vi "Transform Triangle.vi"(6 "Translation Matrix":sgl[][](array[numeric]), 8 "Rotation Z Matrix":sgl[][](array[numeric]), 9 "Rotation Y Matrix":sgl[][](array[numeric]), 10 "Rotation X Matrix":sgl[][](array[numeric]), 11 "Triangle in":T1={"Vertex 1"={"Position"={"x"=0.0, "y"=0.0, "z"=0.0}, "UV"={"u"=0.0, "v"=0.0}, "Colour"=12517256}, "Vertex 2"={"Position"={"x"=0.0, "y"=0.0, "z"=0.0}, "UV"={"u"=0.0, "v"=0.0}, "Colour"=12517256}, "Vertex 3"={"Position"={"x"=0.0, "y"=0.0, "z"=0.0}, "UV"={"u"=0.0, "v"=0.0}, "Colour"=12517256}, "Alpha"=0.0, "Alpha Blending Enabled"=FALSE} {"Vertex 3"."UV"."v" min=0 max=1 step=0.1; "Vertex 3"."UV"."u" min=0 max=1 step=0.1; "Vertex 2"."UV"."v" min=0 max=1 step=0.1; "Vertex 2"."UV"."u" min=0 max=1 step=0.1; "Vertex 1"."UV"."v" min=0 max=1 step=0.1; "Vertex 1"."UV"."u" min=0 max=1 step=0.1}) -> (3 "Triangle out":T1={"Vertex 1"={"Position"={"x"=0.0, "y"=0.0, "z"=0.0}, "UV"={"u"=0.0, "v"=0.0}, "Colour"=12517256}, "Vertex 2"={"Position"={"x"=0.0, "y"=0.0, "z"=0.0}, "UV"={"u"=0.0, "v"=0.0}, "Colour"=12517256}, "Vertex 3"={"Position"={"x"=0.0, "y"=0.0, "z"=0.0}, "UV"={"u"=0.0, "v"=0.0}, "Colour"=12517256}, "Alpha"=0.0, "Alpha Blending Enabled"=FALSE} {"Vertex 3"."UV"."v" min=0 max=1 step=0.1; "Vertex 3"."UV"."u" min=0 max=1 step=0.1; "Vertex 2"."UV"."v" min=0 max=1 step=0.1; "Vertex 2"."UV"."u" min=0 max=1 step=0.1; "Vertex 1"."UV"."v" min=0 max=1 step=0.1; "Vertex 1"."UV"."u" min=0 max=1 step=0.1})   [LabVIEW 2022 SP3, in "3D.lvlib"]
uses:
  3D.lvlib
  Vector 3D.ctl
  Raster/UV.ctl
  Raster/Raster.lvlib
  Vertex.ctl
  Triangle.ctl
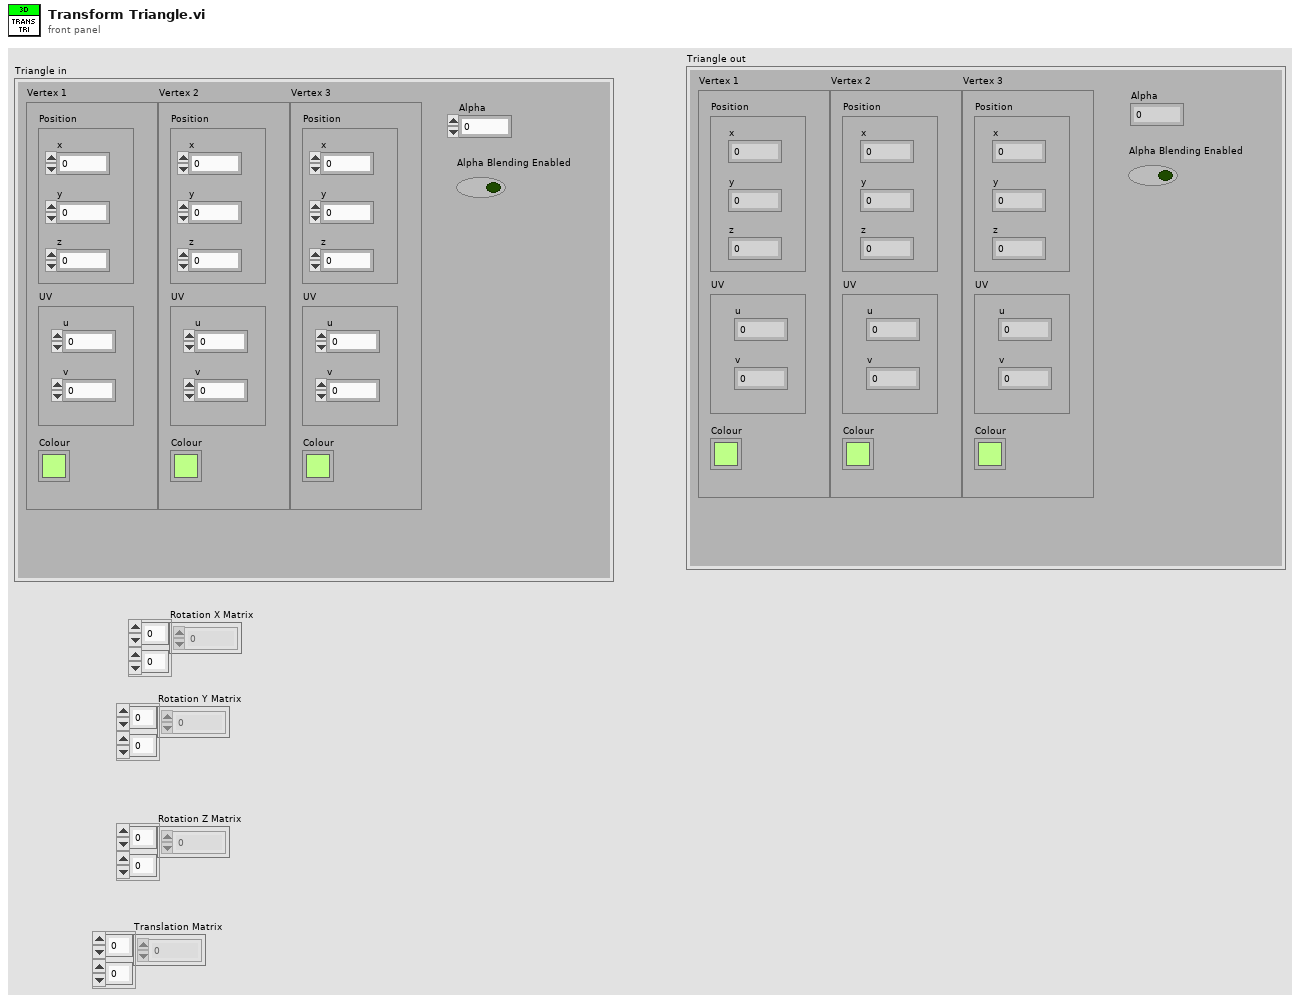
[diagram p1: front panel]
types:
  T1 = typedef "3D.lvlib/Triangle.ctl" = cluster{"Vertex 1":T2, "Vertex 2":T2, "Vertex 3":T2, "Alpha":dbl, "Alpha Blending Enabled":bool}
  T2 = typedef "3D.lvlib/Vertex.ctl" = cluster{"Position":T3, "UV":T4, "Colour":u32}
  T3 = typedef "3D.lvlib/Vector 3D.ctl" = cluster{"x":sgl, "y":sgl, "z":sgl}
  T4 = typedef "Raster.lvlib/UV.ctl" = cluster{"u":sgl, "v":sgl}
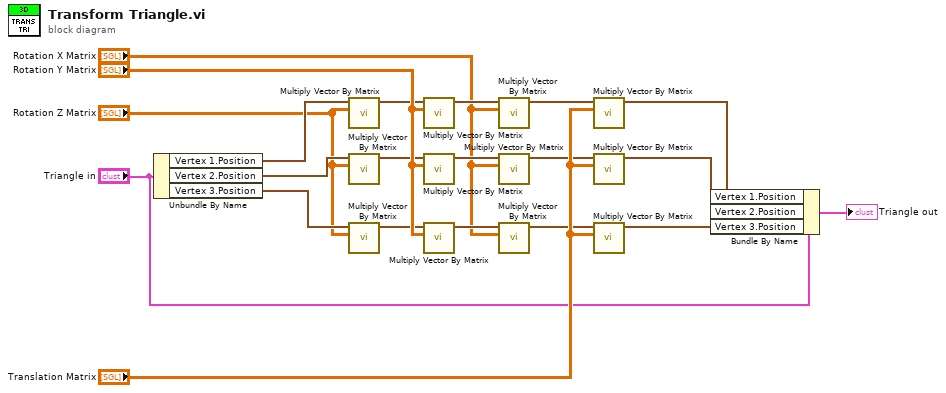
[diagram p0: block diagram]
diagram:
  n1 = Unbundle By Name("Triangle in") -> ("Vertex 1.Position"=w7:T3, "Vertex 2.Position"=w8:T3, "Vertex 3.Position"=w9:T3)
  n2 = call "Multiply Vector By Matrix.vi"("Matrix in"="Rotation Z Matrix", "Vector 3D in"=w7) -> ("Vector 3D out"=w10:T3)  [unwired: 9 in]
  n3 = call "Multiply Vector By Matrix.vi"("Matrix in"="Rotation Z Matrix", "Vector 3D in"=w8) -> ("Vector 3D out"=w12:T3)  [unwired: 9 in]
  n4 = call "Multiply Vector By Matrix.vi"("Matrix in"="Rotation Z Matrix", "Vector 3D in"=w9) -> ("Vector 3D out"=w14:T3)  [unwired: 9 in]
  n5 = call "Multiply Vector By Matrix.vi"("Matrix in"="Rotation Y Matrix", "Vector 3D in"=w10) -> ("Vector 3D out"=w11:T3)  [unwired: 9 in]
  n6 = call "Multiply Vector By Matrix.vi"("Matrix in"="Rotation Y Matrix", "Vector 3D in"=w12) -> ("Vector 3D out"=w13:T3)  [unwired: 9 in]
  n7 = call "Multiply Vector By Matrix.vi"("Matrix in"="Rotation Y Matrix", "Vector 3D in"=w14) -> ("Vector 3D out"=w15:T3)  [unwired: 9 in]
  n8 = call "Multiply Vector By Matrix.vi"("Matrix in"="Rotation X Matrix", "Vector 3D in"=w11) -> ("Vector 3D out"=w4:T3)  [unwired: 9 in]
  n9 = call "Multiply Vector By Matrix.vi"("Matrix in"="Rotation X Matrix", "Vector 3D in"=w13) -> ("Vector 3D out"=w5:T3)  [unwired: 9 in]
  n10 = call "Multiply Vector By Matrix.vi"("Matrix in"="Rotation X Matrix", "Vector 3D in"=w15) -> ("Vector 3D out"=w6:T3)  [unwired: 9 in]
  n11 = call "Multiply Vector By Matrix.vi"("Matrix in"="Translation Matrix", "Vector 3D in"=w4) -> ("Vector 3D out"=w19:T3)  [unwired: 9 in]
  n12 = call "Multiply Vector By Matrix.vi"("Matrix in"="Translation Matrix", "Vector 3D in"=w5) -> ("Vector 3D out"=w20:T3)  [unwired: 9 in]
  n13 = call "Multiply Vector By Matrix.vi"("Matrix in"="Translation Matrix", "Vector 3D in"=w6) -> ("Vector 3D out"=w21:T3)  [unwired: 9 in]
  n14 = Bundle By Name(cluster="Triangle in", "Vertex 1.Position"=w19, "Vertex 2.Position"=w20, "Vertex 3.Position"=w21) -> (→"Triangle out":T1)
